vi "Mark Different Text Red.vi"(5 "reference 2":refnum<vi>, 7 "reference 1":refnum<vi>, 8 "error in (no error)":errorcluster, 10 "String 2":string="<B>item path:</B> C:\\Program Files\\National Instruments\\LabVIEW 8.6\\menus\\Categories\\Data Communication\\sharedvariable.mnu\n\n<B>library path(.lvlib):</B>\n\n<B>use default lvlib palette:</B>False\n\n<B>short name:</B>\n\n<B>place VI contents:False</B>", 11 "String1":string="<B>item path:</B> C:\\Program Files\\National Instruments\\LabVIEW 8.6\\menus\\Categories\\Data Communication\\sharedvariable.mnu\n\n<B>library path(.lvlib):</B>\n\n<B>use default lvlib palette:</B>False\n\n<B>short name:</B>\n\n<B>place VI contents:False</B>") -> (0 "error out":errorcluster)   [LabVIEW 2017]
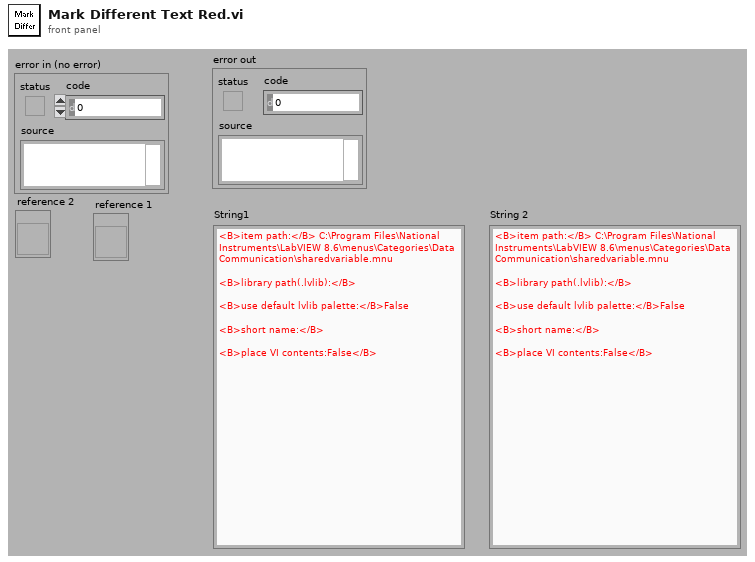
[diagram p1: front panel]
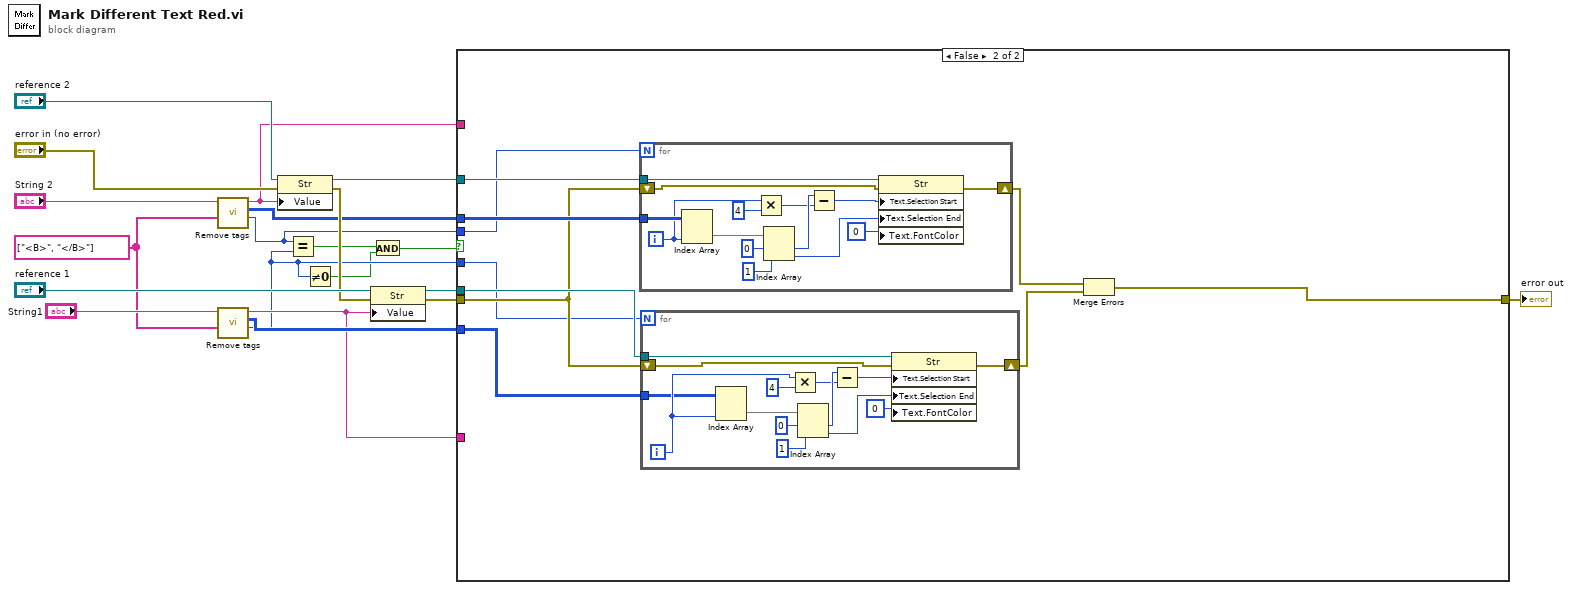
[diagram p0: block diagram]
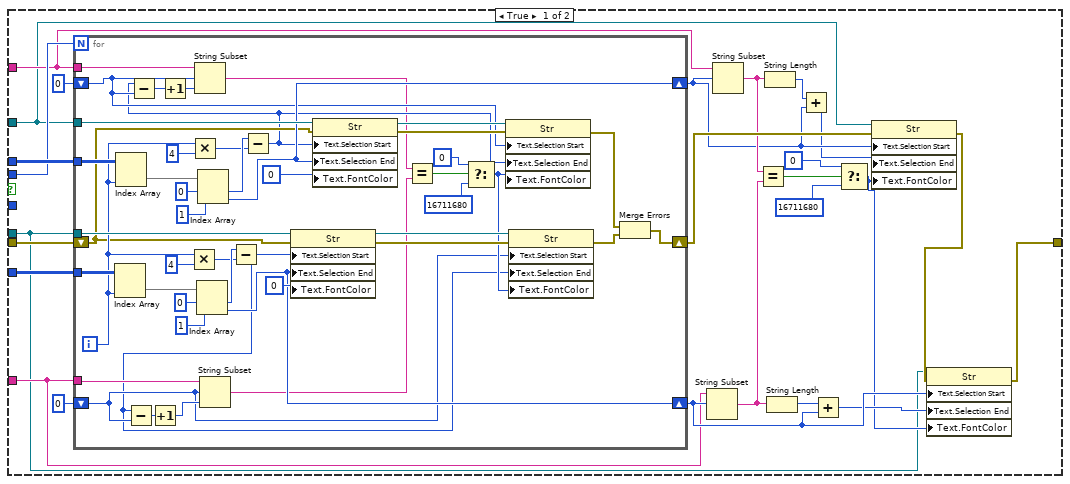
[diagram p2: hidden frame]
diagram:
  w13 = string[] ["<B>", "</B>"] ("operators (none)")
  n1 = call "Remove tags.vi"("separators"=w13, "String in"="String 2") -> ("array size"=w5:i32, "index array"=w9:i32[][], "String out"=w7:string)  [unwired: 7 out]
  n2 = call "Remove tags.vi"("separators"=w13, "String in"="String1") -> ("array size"=w4:i32, "index array"=w19:i32[][], "String out"=w6:string)  [unwired: 7 out]
  n3 = property class="Str"(reference="reference 2", error in="error in (no error)", "Value"=w7) -> (reference out=w8:refnum<vi>, error out=w10:errorcluster)
  n4 = Equal?(x=w5, y=w4) -> (x = y?=w3:bool)
  n5 = Not Equal To 0?(x=w4) -> (x != 0?=w2:bool)
  n6 = property class="Str"(reference="reference 1", error in=w10, "Value"=w6) -> (reference out=w18:refnum<vi>, error out=w16:errorcluster)
  n7 = And(x=w3, y=w2) -> (x .and. y?=w1:bool)
  n8 = case shown="False" w1 {
    tunnel: w19 -> [w45 w96]
    tunnel: w18 -> [w21 w98]
    tunnel: w16 -> [w44 w97]
    tunnel: [w25 w93] -> w15
    tunnel: w9 -> [w43 w100]
    tunnel: w8 -> [w22 w99]
    tunnel: w7 -> [w24 _]
    tunnel: w6 -> [w23 _]
    tunnel: w5 -> [w39 w91]
    tunnel: w4 -> [_ w92]
    frame True {
      n9 = for {
        N: w39 -> [_]
        tunnel: w45 -> [w90]
        tunnel: w21 -> [w83]
        shift-right: [w54] -> w40
        shift-left: w44 -> [w57]
        tunnel: w43 -> [w75]
        tunnel: w22 -> [w72]
        shift-right: [w71] -> w33
        shift-left: 0 -> [w60]
        tunnel: w24 -> [w70]
        tunnel: w23 -> [w67]
        shift-right: [w66] -> w28
        shift-left: 0 -> [w55]
        i -> [w73]
        n10 = Index Array(array=w90, index (col)=w73) -> (element=w89:i32[])  [unwired: 1 in]
        n11 = Index Array(array=w75, index (col)=w73) -> (element=w74:i32[])  [unwired: 1 in]
        n12 = Multiply(x=w73, y=4) -> (x*y=w84:i32)
        n13 = Multiply(x=w73, y=4) -> (x*y=w77:i32)
        n14 = Index Array(array=w89, index #1=0 ("index"), index #2=1 ("index")) -> (element #1=w86:i32, element #2=w66:i32)
        n15 = Index Array(array=w74, index #1=0 ("index"), index #2=1 ("index")) -> (element #1=w79:i32, element #2=w71:i32)
        n16 = Subtract(x=w86, y=w84) -> (x-y=w50:i32)
        n17 = Subtract(x=w50, y=w55) -> (x-y=w69:i32)
        n18 = Increment(x=w69) -> (x+1=w68:i32)
        n19 = String Subset(string=w67, offset (0)=w55, length (rest)=w68) -> (substring=w46:string)
        n20 = Subtract(x=w79, y=w77) -> (x-y=w51:i32)
        n21 = Subtract(x=w51, y=w60) -> (x-y=w49:i32)
        n22 = Increment(x=w49) -> (x+1=w48:i32)
        n23 = String Subset(string=w70, offset (0)=w60, length (rest)=w48) -> (substring=w47:string)
        n24 = property on="Property Node" class="Str"(reference=w83, error in=w57, "Text.Selection Start"=w50, "Text.Selection End"=w66, "Text.FontColor"=u32 0 ("Text.Font:Color")) -> (reference out=w59:refnum<vi>, error out=w58:errorcluster)
        n25 = property on="Property Node" class="Str"(reference=w72, error in=w57, "Text.Selection Start"=w51, "Text.Selection End"=w71, "Text.FontColor"=u32 0 ("Text.Font:Color")) -> (reference out=w62:refnum<vi>, error out=w61:errorcluster)
        n26 = Equal?(x=w47, y=w46) -> (x = y?=w65:bool)
        n27 = Select(t=0, s=w65, f=16711680) -> (s? t:f=w56:i32)
        n28 = property class="Str"(reference=w62, error in=w61, "Text.Selection Start"=w60, "Text.Selection End"=w51, "Text.FontColor"=w56) -> (error out=w53:errorcluster)  [unwired: 1 out]
        n29 = property class="Str"(reference=w59, error in=w58, "Text.Selection Start"=w55, "Text.Selection End"=w50, "Text.FontColor"=w56) -> (error out=w52:errorcluster)  [unwired: 1 out]
        n30 = Merge Errors(w53, w52) -> (w54:errorcluster)
      }
      n31 = String Subset(string=w23, offset (0)=w28) -> (substring=w30:string)  [unwired: 1 out]
      n32 = String Subset(string=w24, offset (0)=w33) -> (substring=w35:string)  [unwired: 1 out]
      n33 = Equal?(x=w35, y=w30) -> (x = y?=w38:bool)
      n34 = String Length(string=w35) -> (length=w34:i32)
      n35 = String Length(string=w30) -> (length=w29:i32)
      n36 = Add(x=w34, y=w33) -> (x+y=w32:i32)
      n37 = Add(x=w29, y=w28) -> (x+y=w27:i32)
      n38 = Select(t=0, s=w38, f=16711680) -> (s? t:f=w26:i32)
      n39 = property class="Str"(reference=w22, error in=w40, "Text.Selection Start"=w33, "Text.Selection End"=w32, "Text.FontColor"=w26) -> (error out=w31:errorcluster)  [unwired: 1 out]
      n40 = property class="Str"(reference=w21, error in=w31, "Text.Selection Start"=w28, "Text.Selection End"=w27, "Text.FontColor"=w26) -> (error out=w25:errorcluster)  [unwired: 1 out]
    }
    frame False {
      n41 = for {
        N: w91 -> [_]
        shift-right: [w116] -> w95
        shift-left: w97 -> [w117]
        tunnel: w100 -> [w122]
        tunnel: w99 -> [w120]
        i -> [w115]
        n42 = Index Array(array=w122, index (col)=w115) -> (element=w121:i32[])  [unwired: 1 in]
        n43 = Multiply(x=w115, y=4) -> (x*y=w124:i32)
        n44 = Index Array(array=w121, index #1=0 ("index"), index #2=1 ("index")) -> (element #1=w126:i32, element #2=w119:i32)
        n45 = Subtract(x=w126, y=w124) -> (x-y=w118:i32)
        n46 = property on="Property Node" class="Str"(reference=w120, error in=w117, "Text.Selection Start"=w118, "Text.Selection End"=w119, "Text.FontColor"=u32 0 ("Text.Font:Color")) -> (error out=w116:errorcluster)  [unwired: 1 out]
      }
      n47 = for {
        N: w92 -> [_]
        tunnel: w98 -> [w105]
        shift-right: [w102] -> w94
        shift-left: w97 -> [w103]
        tunnel: w96 -> [w101]
        i -> [w104]
        n48 = Index Array(array=w101, index (col)=w104) -> (element=w114:i32[])  [unwired: 1 in]
        n49 = Multiply(x=w104, y=4) -> (x*y=w109:i32)
        n50 = Index Array(array=w114, index #1=0 ("index"), index #2=1 ("index")) -> (element #1=w111:i32, element #2=w107:i32)
        n51 = Subtract(x=w111, y=w109) -> (x-y=w106:i32)
        n52 = property on="Property Node" class="Str"(reference=w105, error in=w103, "Text.Selection Start"=w106, "Text.Selection End"=w107, "Text.FontColor"=u32 0 ("Text.Font:Color")) -> (error out=w102:errorcluster)  [unwired: 1 out]
      }
      n53 = Merge Errors(w95, w94) -> (w93:errorcluster)
    }
  }
  "error out" <- w15
